vi "Control Selector.vi"(11 "Controller Diagram":T1) -> (3 "String":string)   [LabVIEW 2015]
uses:
  Common Code/Controller Diagram.ctl
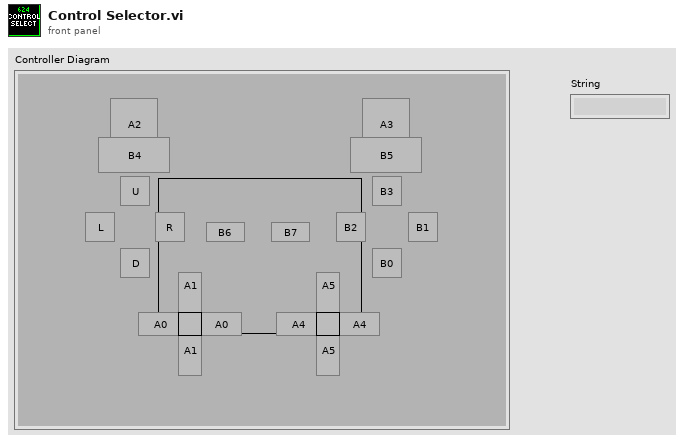
[diagram p1: front panel]
types:
  T1 = typedef "Controller Diagram.ctl" = cluster{"Button 4":bool, "Button 5":bool, "Axis 2":bool, "Axis 3":bool, "Button 6":bool, "Button 7":bool, "Button 0":bool, "Button 1":bool, "Button 2":bool, "Button 3":bool, "POV Down":bool, "POV Right":bool, "POV Left":bool, "POV Up":bool, "Axis 1":bool, "Axis 0":bool, "Axis 4":bool, "Axis 5":bool}
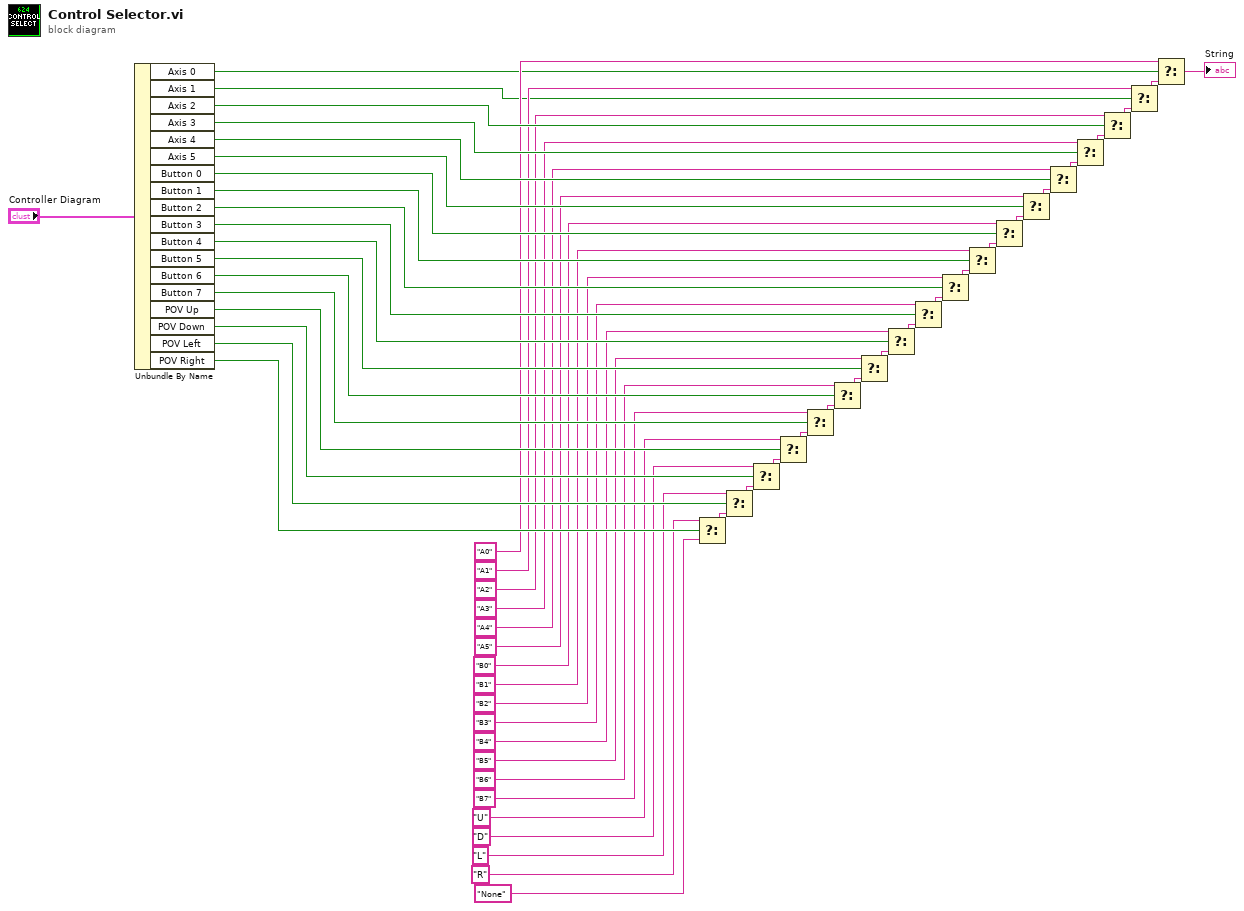
[diagram p0: block diagram]
diagram:
  n1 = Unbundle By Name("Controller Diagram") -> ("Axis 0"=w3:bool, "Axis 1"=w2:bool, "Axis 2"=w56:bool, "Axis 3"=w55:bool, "Axis 4"=w54:bool, "Axis 5"=w42:bool, "Button 0"=w53:bool, "Button 1"=w52:bool, "Button 2"=w51:bool, "Button 3"=w50:bool, "Button 4"=w49:bool, "Button 5"=w48:bool, "Button 6"=w47:bool, "Button 7"=w41:bool, "POV Up"=w46:bool, "POV Down"=w45:bool, "POV Left"=w44:bool, "POV Right"=w43:bool)
  n2 = Select(t="R", s=w43, f="None") -> (s? t:f=w40:string)
  n3 = Select(t="L", s=w44, f=w40) -> (s? t:f=w39:string)
  n4 = Select(t="D", s=w45, f=w39) -> (s? t:f=w38:string)
  n5 = Select(t="U", s=w46, f=w38) -> (s? t:f=w37:string)
  n6 = Select(t="B7", s=w41, f=w37) -> (s? t:f=w36:string)
  n7 = Select(t="B6", s=w47, f=w36) -> (s? t:f=w35:string)
  n8 = Select(t="B5", s=w48, f=w35) -> (s? t:f=w34:string)
  n9 = Select(t="B4", s=w49, f=w34) -> (s? t:f=w33:string)
  n10 = Select(t="B3", s=w50, f=w33) -> (s? t:f=w32:string)
  n11 = Select(t="B2", s=w51, f=w32) -> (s? t:f=w31:string)
  n12 = Select(t="B1", s=w52, f=w31) -> (s? t:f=w30:string)
  n13 = Select(t="B0", s=w53, f=w30) -> (s? t:f=w29:string)
  n14 = Select(t="A5", s=w42, f=w29) -> (s? t:f=w28:string)
  n15 = Select(t="A4", s=w54, f=w28) -> (s? t:f=w27:string)
  n16 = Select(t="A3", s=w55, f=w27) -> (s? t:f=w26:string)
  n17 = Select(t="A2", s=w56, f=w26) -> (s? t:f=w25:string)
  n18 = Select(t="A1", s=w2, f=w25) -> (s? t:f=w24:string)
  n19 = Select(t="A0", s=w3, f=w24) -> (s? t:f=→"String":string)
